vi "Untitled 13.vi"(0 "connection reference 2":T1, 2 "report in":refnum<class "NI_report.lvclass">, 5 "error in (no error) 2":errorcluster) -> (14 "connection reference":T1, 16 "error out":errorcluster, 17 "report out":refnum<class "NI_report.lvclass">, 19 "error out 2":errorcluster)   [LabVIEW 2012]
uses:
  <vilib>/addons/database/Connection.llb/Conn ObjectReference.ctl
  <vilib>/Utility/NIReport.llb/NI_report.lvclass
  <vilib>/addons/database/Auxilliary.llb/DB Tools Cursor Type.ctl
  <vilib>/addons/database/Connection.llb/Conn Execute.vi
  <vilib>/addons/database/Recordset.llb/Rec Fetch String Data (R).vi
  <vilib>/addons/database/Recordset.llb/Rec Fetch Integer Data (R).vi
  <vilib>/addons/database/Recordset.llb/Rec Destroy - Connection.vi
  <vilib>/addons/database/NI_Database_API.lvlib
  <vilib>/Utility/NIReport.llb/Excel/NI_Excel.lvclass
panel:
  in  "start (0, 0)":cluster{"start row":i32, "start column":i32}
  in  "start row":i32
  in  "string":string
  in  "error in (no error)":errorcluster
  out "concatenated string":string
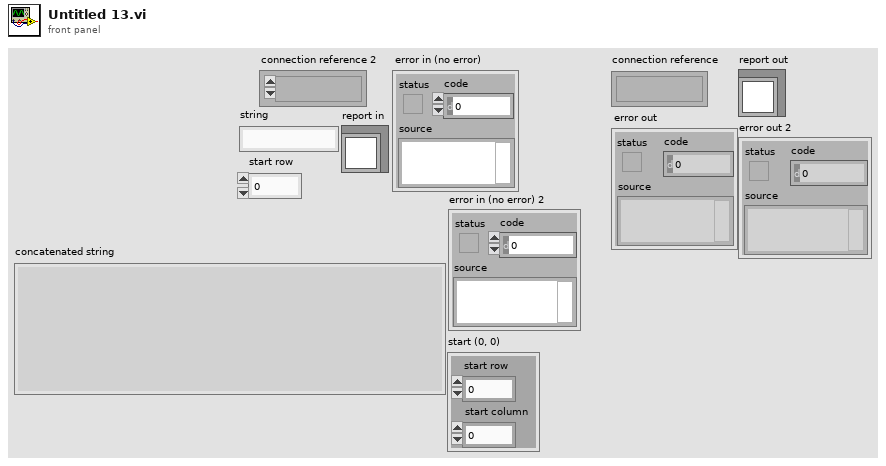
[diagram p1: front panel]
types:
  T1 = typedef "NI_Database_API.lvlib/Conn ObjectReference.ctl" = refnum<k1>
  T2 = typedef "NI_Database_API.lvlib/DB Tools Cursor Type.ctl" = enum16{"forward-only", "keyset", "dynamic", "static"}
  T3 = typedef "NI_Database_API.lvlib/Rec ObjectReference.ctl" = refnum<k1>
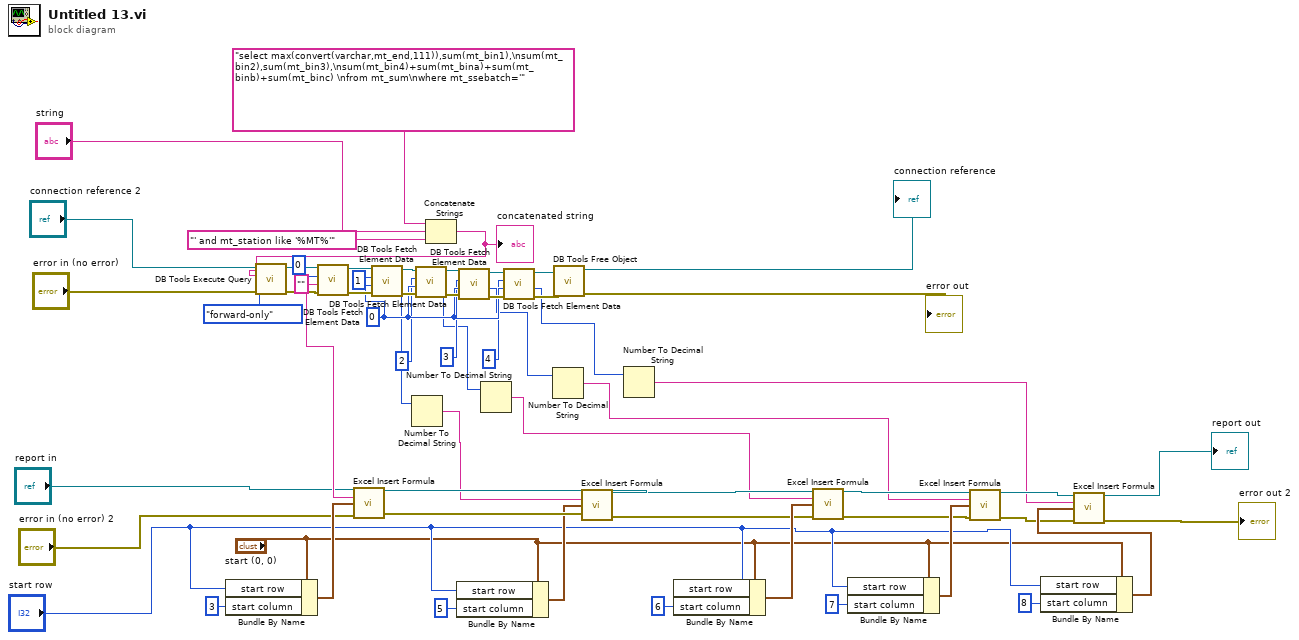
[diagram p0: block diagram]
diagram:
  w43 = 0
  n1 = Bundle By Name(cluster="start (0, 0)", "start row"="start row", "start column"=3) -> (w38:cluster{"start row":i32, "start column":i32})
  n2 = Concatenate Strings("select max(convert(varchar,mt_end,111)),sum(mt_bin1),\nsum(mt_bin2),sum(mt_bin3),\nsum(mt_bin4)+sum(mt_bina)+sum(mt_binb)+sum(mt_binc) \nfrom mt_sum\nwhere mt_ssebatch='", "string", "' and mt_station like '%MT%'" ("string")) -> (w59:string)
  "concatenated string" <- w59
  n3 = call-poly <vilib>:"DB Tools Execute Query.vi"("error in (no error)"="error in (no error)", "cursor type"=DB_Tools_Cursor_Type."forward-only", "SQL query"=w59, "connection reference"="connection reference 2") -> ("error out"=w56:errorcluster, "recordset reference"=w57:T3)  [unwired: 4 in]
  n4 = call-poly <vilib>:"DB Tools Fetch Element Data.vi"("error in (no error)"=w56, "type"="", "column index"=0, "recordset reference"=w57) -> ("error out"=w52:errorcluster, "data"=w37:string, "recordset reference out"=w53:T3)  [unwired: 3 in]
  n5 = call <vilib>:"Excel Insert Formula.vi"("report in"="report in", "formula"=w37, "start (0, 0)"=w38, "error in (no error)"="error in (no error) 2") -> ("report out"=w35:refnum<class "NI_report.lvclass">, "error out"=w34:errorcluster)  [unwired: 10 in]
  n6 = call-poly <vilib>:"DB Tools Fetch Element Data.vi"("error in (no error)"=w52, "type"=w43, "column index"=1, "recordset reference"=w53) -> ("error out"=w47:errorcluster, "data"=w32:i32, "recordset reference out"=w51:T3)  [unwired: 3 in]
  n7 = Number To Decimal String(number=w32) -> (decimal integer string=w31:string)  [unwired: 1 in]
  n8 = call-poly <vilib>:"DB Tools Fetch Element Data.vi"("error in (no error)"=w47, "type"=w43, "column index"=2, "recordset reference"=w51) -> ("error out"=w46:errorcluster, "data"=w25:i32, "recordset reference out"=w50:T3)  [unwired: 3 in]
  n9 = Bundle By Name(cluster="start (0, 0)", "start row"="start row", "start column"=5) -> (w30:cluster{"start row":i32, "start column":i32})
  n10 = call-poly <vilib>:"DB Tools Fetch Element Data.vi"("error in (no error)"=w46, "type"=w43, "column index"=3, "recordset reference"=w50) -> ("error out"=w45:errorcluster, "data"=w23:i32, "recordset reference out"=w49:T3)  [unwired: 3 in]
  n11 = Number To Decimal String(number=w25) -> (decimal integer string=w24:string)  [unwired: 1 in]
  n12 = call-poly <vilib>:"DB Tools Fetch Element Data.vi"("error in (no error)"=w45, "type"=w43, "column index"=4, "recordset reference"=w49) -> ("error out"=w44:errorcluster, "data"=w22:i32, "recordset reference out"=w48:T3)  [unwired: 3 in]
  n13 = Number To Decimal String(number=w23) -> (decimal integer string=w13:string)  [unwired: 1 in]
  n14 = call-poly <vilib>:"DB Tools Free Object.vi"("error in (no error)"=w44, "recordset reference"=w48) -> ("error out"=→"error out":errorcluster, "connection reference"=→"connection reference":T1)  [unwired: 8 in]
  n15 = call <vilib>:"Excel Insert Formula.vi"("report in"=w35, "formula"=w31, "start (0, 0)"=w30, "error in (no error)"=w34) -> ("report out"=w26:refnum<class "NI_report.lvclass">, "error out"=w28:errorcluster)  [unwired: 10 in]
  n16 = Number To Decimal String(number=w22) -> (decimal integer string=w12:string)  [unwired: 1 in]
  n17 = Bundle By Name(cluster="start (0, 0)", "start row"="start row", "start column"=6) -> (w29:cluster{"start row":i32, "start column":i32})
  n18 = call <vilib>:"Excel Insert Formula.vi"("report in"=w26, "formula"=w24, "start (0, 0)"=w29, "error in (no error)"=w28) -> ("report out"=w17:refnum<class "NI_report.lvclass">, "error out"=w15:errorcluster)  [unwired: 10 in]
  n19 = Bundle By Name(cluster="start (0, 0)", "start row"="start row", "start column"=7) -> (w19:cluster{"start row":i32, "start column":i32})
  n20 = call <vilib>:"Excel Insert Formula.vi"("report in"=w17, "formula"=w13, "start (0, 0)"=w19, "error in (no error)"=w15) -> ("report out"=w16:refnum<class "NI_report.lvclass">, "error out"=w14:errorcluster)  [unwired: 10 in]
  n21 = Bundle By Name(cluster="start (0, 0)", "start row"="start row", "start column"=8) -> (w18:cluster{"start row":i32, "start column":i32})
  n22 = call <vilib>:"Excel Insert Formula.vi"("report in"=w16, "formula"=w12, "start (0, 0)"=w18, "error in (no error)"=w14) -> ("report out"=→"report out":refnum<class "NI_report.lvclass">, "error out"=→"error out 2":errorcluster)  [unwired: 10 in]
